vi "数据存储接口.vi"(5 "质控参数设置":T1, 7 "数据标记表":string, 9 "SN":string, 10 "数据存储模式":enum16{"水样测试", "标样核查", "跨度核查", "零点核查", "加标回收"}(ring), 11 "测量数据区":T3) -> (3 "data输出":T2)   [LabVIEW 2016, in "斯坦道总磷总氮V2.lvlib"]
panel:
  # "跨度值"
  # "零点核查标准液浓度"
  # "跨度核查标准液浓度"
  # "标样核查标准液浓度"
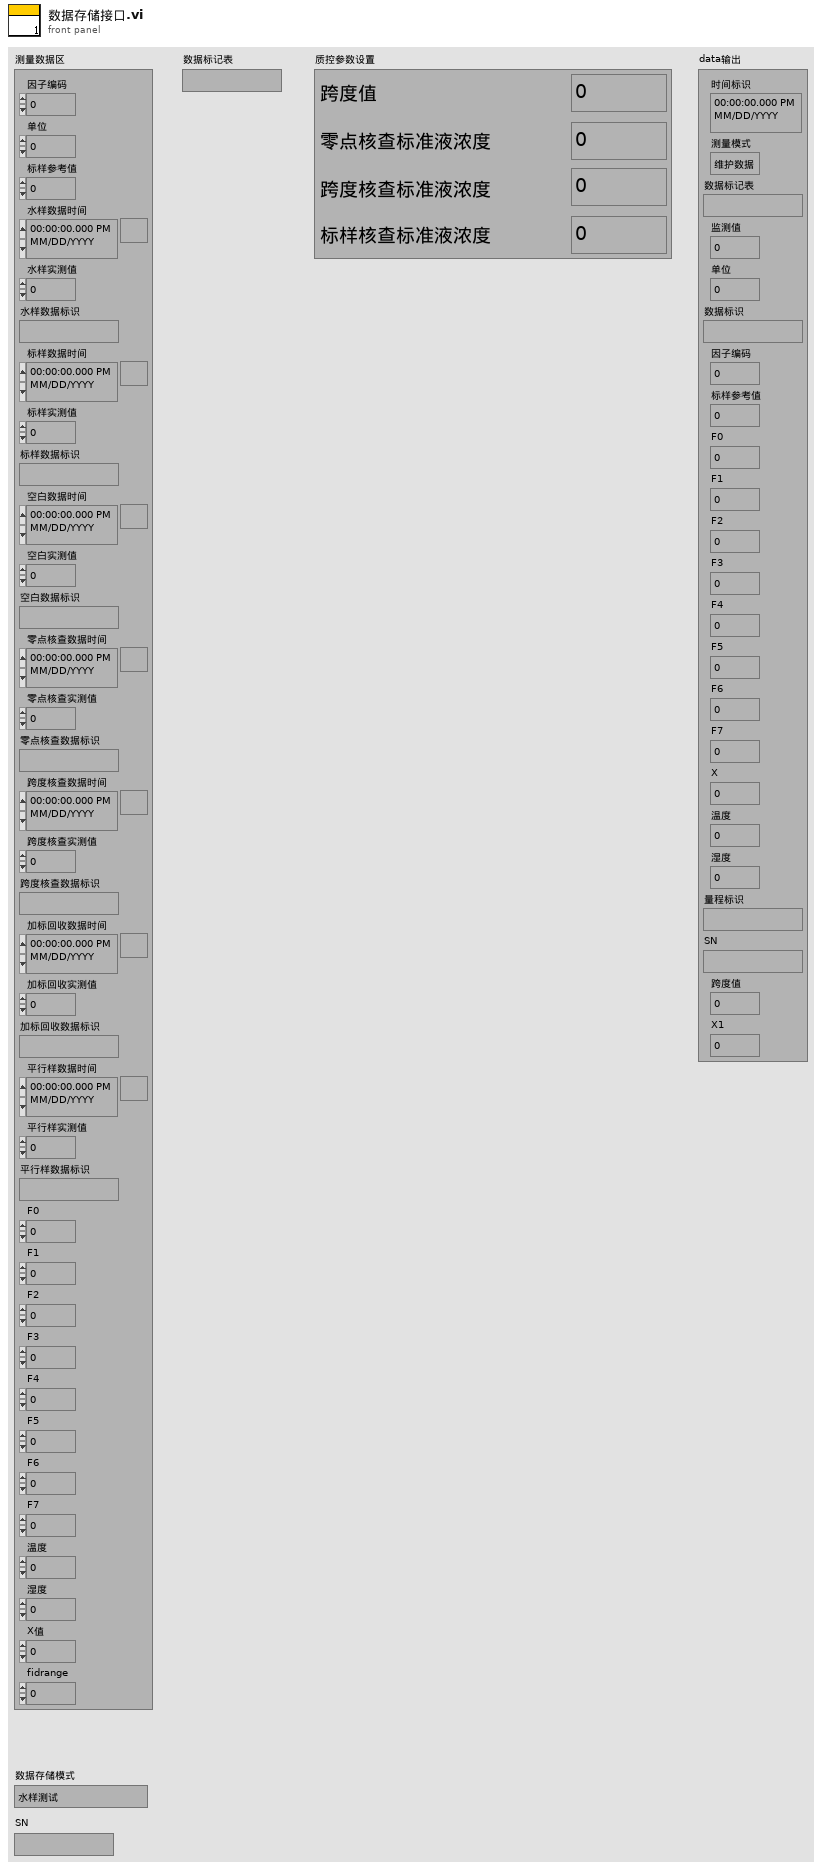
[diagram p1: front panel]
types:
  T1 = cluster{"跨度值":dbl, "零点标准液浓度":dbl, "跨度标准液浓度":dbl, "标准液标准浓度":dbl}
  T2 = cluster{"时间标识":timestamp, "测量模式":enum16{"维护数据", "水样测试", "标样核查", "零点核查", "跨度核查", "空白测试", "平行样测试", "加标回收", "空白校准", "标样校准", "初始化（清洗）", "快捷测试"}, "数据标记表":string, "监测值":sgl, "单位":u16, "数据标识":string, "因子编码":u32, "标样参考值":sgl, "F0":sgl, "F1":sgl, "F2":sgl, "F3":sgl, "F4":sgl, "F5":sgl, "F6":sgl, "F7":sgl, "X":sgl, "温度":sgl, "湿度":sgl, "量程标识":string, "SN":string, "跨度值":sgl, "X1":sgl}
  T3 = cluster{"因子编码":u32, "单位":u16, "标样参考值":sgl, "水样数据时间":timestamp, "水样实测值":sgl, "水样数据标识":string, "标样数据时间":timestamp, "标样实测值":sgl, "标样数据标识":string, "空白数据时间":timestamp, "空白实测值":sgl, "空白数据标识":string, "零点核查数据时间":timestamp, "零点核查实测值":sgl, "零点核查数据标识":string, "跨度核查数据时间":timestamp, "跨度核查实测值":sgl, "跨度核查数据标识":string, "加标回收数据时间":timestamp, "加标回收实测值":sgl, "加标回收数据标识":string, "平行样数据时间":timestamp, "平行样实测值":sgl, "平行样数据标识":string, "F0":sgl, "F1":sgl, "F2":sgl, "F3":sgl, "F4":sgl, "F5":sgl, "F6":sgl, "F7":sgl, "温度":sgl, "湿度":sgl, "X值":sgl, "fidrange":u16}
  T4 = enum16{"维护数据", "水样测试", "标样核查", "零点核查", "跨度核查", "空白测试", "平行样测试", "加标回收", "空白校准", "标样校准", "初始化（清洗）", "快捷测试"}
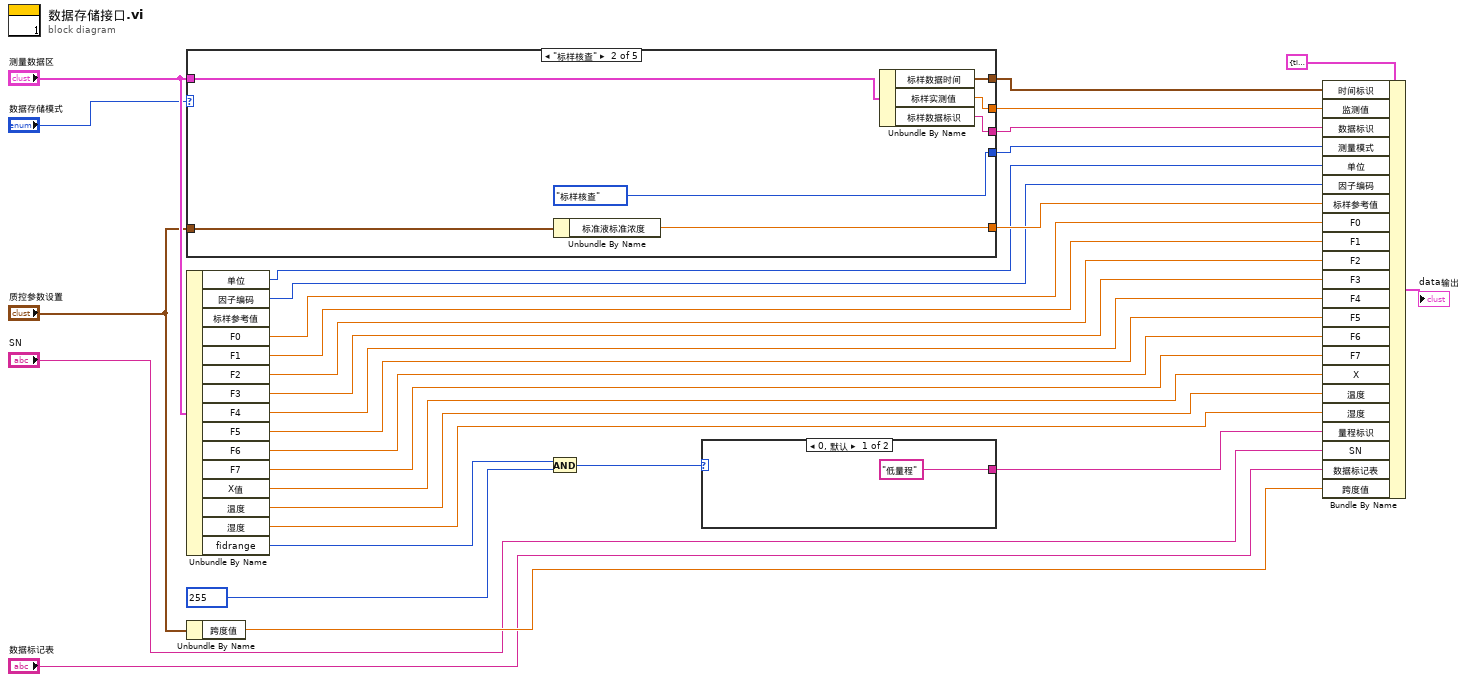
[diagram p0: block diagram]
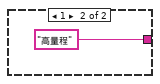
[diagram p2: hidden frame]
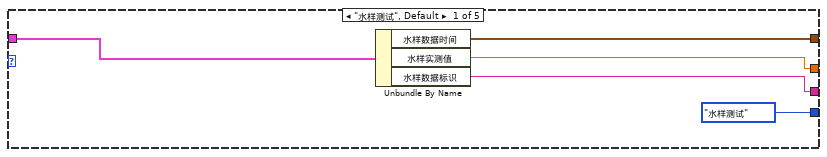
[diagram p3: hidden frame]
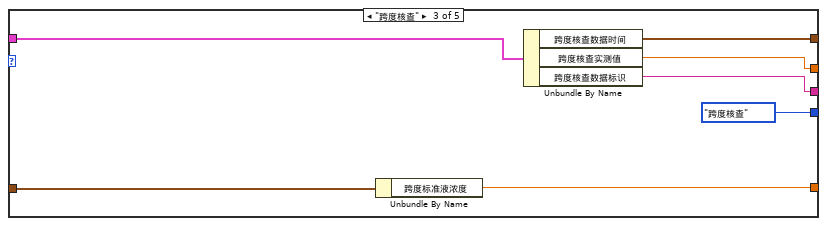
[diagram p4: hidden frame]
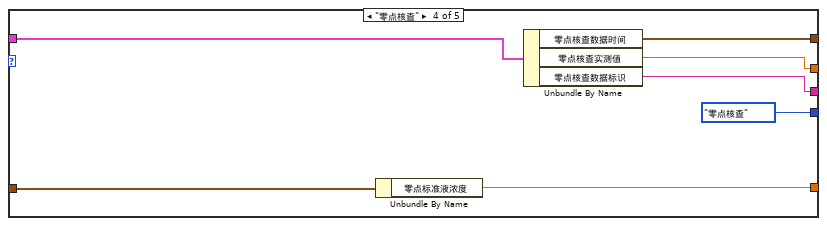
[diagram p5: hidden frame]
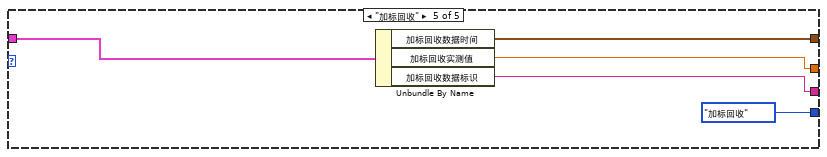
[diagram p6: hidden frame]
diagram:
  n1 = case shown="\"标样核查\"" "数据存储模式" {
    tunnel: "测量数据区" -> [w35 w42 w49 w56 w61]
    tunnel: [w34 w41 w48 w55 w60] -> w18
    tunnel: [w33 w40 w47 w54 w59] -> w17
    tunnel: [w32 w39 w46 w53 w58] -> w16
    tunnel: [T4."水样测试" ("测量模式") T4."标样核查" ("测量模式") T4."跨度核查" ("测量模式") T4."零点核查" ("测量模式") T4."加标回收" ("测量模式")] -> w27
    tunnel: "质控参数设置" -> [_ w38 w45 w52 _]
    tunnel: [_ w37 w44 w51 _] -> w20
    frame "水样测试", Default {
      n2 = Unbundle By Name(w35) -> ("水样数据时间"=w34:timestamp, "水样实测值"=w33:sgl, "水样数据标识"=w32:string)
    }
    frame "标样核查" {
      n3 = Unbundle By Name(w38) -> ("标准液标准浓度"=w37:dbl)
      n4 = Unbundle By Name(w42) -> ("标样数据时间"=w41:timestamp, "标样实测值"=w40:sgl, "标样数据标识"=w39:string)
    }
    frame "跨度核查" {
      n5 = Unbundle By Name(w45) -> ("跨度标准液浓度"=w44:dbl)
      n6 = Unbundle By Name(w49) -> ("跨度核查数据时间"=w48:timestamp, "跨度核查实测值"=w47:sgl, "跨度核查数据标识"=w46:string)
    }
    frame "零点核查" {
      n7 = Unbundle By Name(w52) -> ("零点标准液浓度"=w51:dbl)
      n8 = Unbundle By Name(w56) -> ("零点核查数据时间"=w55:timestamp, "零点核查实测值"=w54:sgl, "零点核查数据标识"=w53:string)
    }
    frame "加标回收" {
      n9 = Unbundle By Name(w61) -> ("加标回收数据时间"=w60:timestamp, "加标回收实测值"=w59:sgl, "加标回收数据标识"=w58:string)
    }
  }
  n10 = Unbundle By Name("测量数据区") -> ("单位"=w3:u16, "因子编码"=w4:u32, "F0"=w5:sgl, "F1"=w6:sgl, "F2"=w7:sgl, "F3"=w8:sgl, "F4"=w9:sgl, "F5"=w10:sgl, "F6"=w11:sgl, "F7"=w12:sgl, "X值"=w13:sgl, "温度"=w14:sgl, "湿度"=w15:sgl, "fidrange"=w21:u16)  [unwired: 1 out]
  n11 = Unbundle By Name("质控参数设置") -> ("跨度值"=w29:dbl)
  n12 = And(x=w21, y=u16 255) -> (x .and. y?=w23:u16)
  n13 = case shown="0, 默认" w23 {
    tunnel: ["低量程" ("格式字符串") "高量程" ("格式字符串")] -> w24
    frame 0, Default {
    }
    frame 1 {
    }
  }
  n14 = Bundle By Name(cluster=T2 {"时间标识"=timestamp(0 s since 1904-01-01), "测量模式"=enum."维护数据", "数据标记表"="", "监测值"=0.0, "单位"=0, "数据标识"="", "因子编码"=0, "标样参考值"=0.0, "F0"=0.0, "F1"=0.0, "F2"=0.0, "F3"=0.0, "F4"=0.0, "F5"=0.0, "F6"=0.0, "F7"=0.0, "X"=0.0, "温度"=0.0, "湿度"=0.0, "量程标识"="", "SN"="", "跨度值"=0.0, "X1"=0.0} ("data输入"), "时间标识"=w18, "监测值"=w17, "数据标识"=w16, "测量模式"=w27, "单位"=w3, "因子编码"=w4, "标样参考值"=w20, "F0"=w5, "F1"=w6, "F2"=w7, "F3"=w8, "F4"=w9, "F5"=w10, "F6"=w11, "F7"=w12, "X"=w13, "温度"=w14, "湿度"=w15, "量程标识"=w24, "SN"="SN", "数据标记表"="数据标记表", "跨度值"=w29) -> (→"data输出":T2)
